vi "Init.vi"(10 "History Length":u32=100, 11 "Digital Waveform Chart in":refnum<class "Digital Waveform Chart.lvclass">) -> (3 "Digital Waveform Chart out":refnum<class "Digital Waveform Chart.lvclass">)   [LabVIEW 2024, in "Digital Waveform Chart.lvclass"]
uses:
  Digital Waveform Chart.lvclass
  Digital Waveform Chart.lvclass/Digital Waveform Chart.ctl
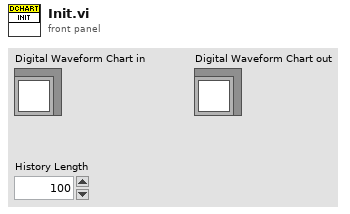
[diagram p1: front panel]
types:
  T1 = cluster{"buffer":digitalwaveform[], "index of latest":i32, "count of added":i32}[]
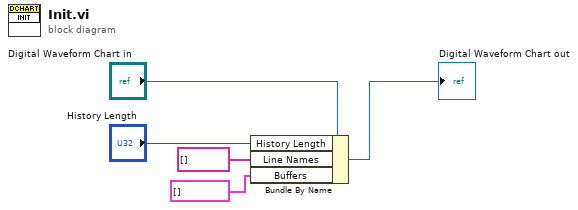
[diagram p0: block diagram]
diagram:
  n1 = Bundle By Name(cluster="Digital Waveform Chart in", "History Length"="History Length", "Line Names"=string[] [], "Buffers"=T1 []) -> (→"Digital Waveform Chart out":refnum<class "Digital Waveform Chart.lvclass">)
